vi "niRFUtil FTW Generate VBW FIR Filter.vi"(10 "Sampling Period (sec)":dbl format="%^.2e", 11 "VBW (Hz)":dbl=30000.0 format="%^.2e") -> (3 "Filter":T1={"x0"=-2.777777777777778e-06, "dx"=4.6296296296296297e-07, "y"=[]} {"y" min=0 max=127 format="%.2f"; "dx" format="%^.2e"; "x0" format="%^.2e"})   [LabVIEW 2015, in "niRFUtil.lvlib"]
uses:
  niRFUtil.lvlib
  Includes/niRFUtil INC Real Waveform.ctl
  Includes/niRFUtil INC Real Array.ctl
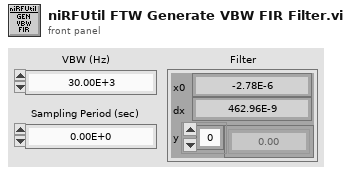
[diagram p1: front panel]
types:
  T1 = typedef "niRFUtil.lvlib/niRFUtil INC Real Waveform.ctl" = cluster{"x0":dbl, "dx":dbl, "y":T2}
  T2 = typedef "niRFUtil.lvlib/niRFUtil INC Real Array.ctl" = sgl[]
  T3 = cluster{"VBW (Hz)":dbl, "Sampling Period (sec)":dbl}
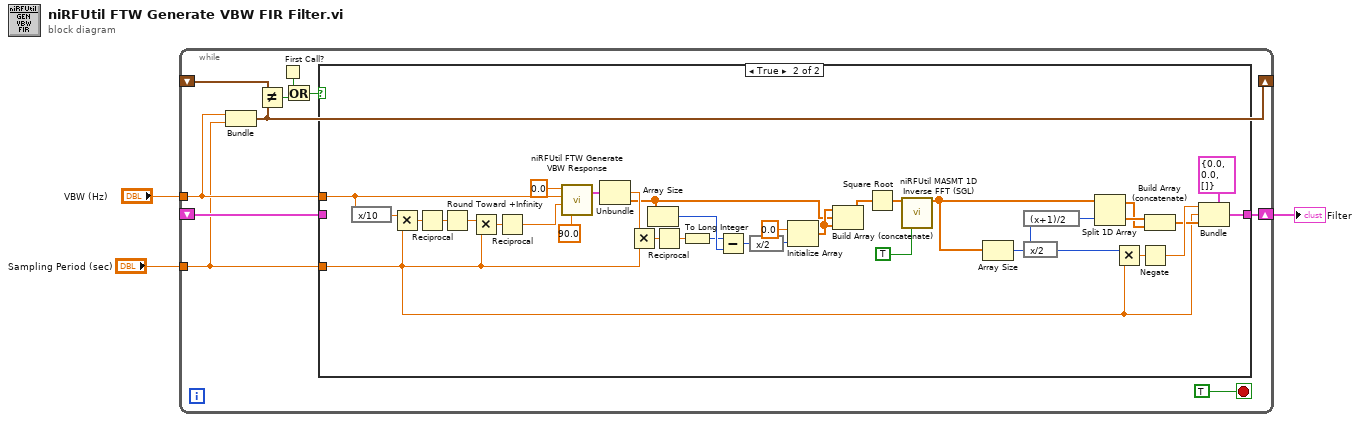
[diagram p0: block diagram]
diagram:
  n1 = while {
    tunnel: "VBW (Hz)" -> [w10]
    tunnel: "Sampling Period (sec)" -> [w9]
    shift-right: [w13] -> w1
    shift-left: _ -> [w11]
    shift-right: [w7] -> _
    shift-left: _ -> [w8]
    stop <- TRUE stop-if-true
    n2 = Bundle("VBW (Hz)"=w10, "Sampling Period (sec)"=w9) -> (w7:T3)  [unwired: 1 out]
    n3 = Not Equal?(x=w8, y=w7) -> (x != y?=w6:bool)
    n4 = First Call?() -> (First Call?: T/F=w4:bool)
    n5 = Or(x=w4, y=w6) -> (x .or. y?=w5:bool)
    n6 = case shown="True" w5 {
      tunnel: [w14 w49] -> w13
      tunnel: w9 -> [_ w28]
      tunnel: w10 -> [_ w36]
      tunnel: w11 -> [w14 _]
      frame False {
      }
      frame True {
        n7 = expression code="x/10"(w36) -> (w35:dbl)
        n8 = Multiply(x=w35, y=w28) -> (x*y=w34:dbl)
        n9 = Reciprocal(x=w34) -> (1/x=w33:dbl)
        n10 = Round Toward +Infinity(x=w33) -> (ceil(x): smallest int >= x=w32:dbl)
        n11 = Multiply(x=w32, y=w28) -> (x*y=w31:dbl)
        n12 = Reciprocal(x=w31) -> (1/x=w30:dbl)
        n13 = call "niRFUtil FTW Generate VBW Response.vi"("Minimum Selectivity (dB)"=90.0 ("Minimum Selectivity, dB"), "df (Hz)"=w30, "VBW (Hz)"=w36, "Center Frequency (Hz)"=0.0 ("Center Frequency, Hz")) -> ("Filter Power Response"=w47:T1)
        n14 = Unbundle(w47) -> ("dx"=w29:dbl, "y"=w20:T2)  [unwired: 1 out]
        n15 = Multiply(x=w29, y=w28) -> (x*y=w27:dbl)
        n16 = Array Size(array=w20) -> (size(s)=w25:i32)
        n17 = Reciprocal(x=w27) -> (1/x=w26:dbl)
        n18 = To Long Integer(number=w26) -> (32bit integer=w23:i32)
        n19 = Subtract(x=w23, y=w25) -> (x-y=w24:i32)
        n20 = expression code="x/2"(w24) -> (w22:i32)
        n21 = Initialize Array(sgl 0.0 ("element"), w22) -> (w21:sgl[])
        n22 = Build Array (concatenate)(w21, w20, w21) -> (w19:T2)
        n23 = Square Root(x=w19) -> (sqrt(x)=w38:T2)
        n24 = call "niRFUtil MASMT 1D Inverse FFT (SGL).vi"("FFT {X}"=w38, "shift?"=TRUE) -> ("X"=w16:sgl[])  [unwired: 12 in, 1 out]
        n25 = Array Size(array=w16) -> (size(s)=w40:i32)
        n26 = expression code="(x+1)/2"(w40) -> (w39:i32)
        n27 = expression code="x/2"(w40) -> (w41:i32)
        n28 = Split 1D Array(array=w16, index=w39) -> (first subarray=w42:sgl[], second subarray=w43:sgl[])
        n29 = Multiply(x=w41, y=w28) -> (x*y=w46:dbl)
        n30 = Negate(x=w46) -> (-x=w45:dbl)
        n31 = Build Array (concatenate)(w43, w42) -> (w37:sgl[])
        n32 = Bundle(cluster=T1 {"x0"=0.0, "dx"=0.0, "y"=[]} ("Filter"), "x0"=w45, "dx"=w28, "y"=w37) -> (w49:T1)
      }
    }
  }
  "Filter" <- w1
